vi "ListSharedResources.vi"(7 "exact name? (F: regex)":bool caption="exact", 8 "error in (no error)":errorcluster, 10 "Filter (regex|name)":string caption="Filter", 11 "SMO in":refnum<class "SMO.lvclass">) -> (0 "error out":errorcluster, 1 "resources found?":bool, 2 "Shared Resources":refnum<class "SMO.lvclass">[](array[class]), 3 "SMO out":refnum<class "SMO.lvclass">)   [LabVIEW 2021, in "smo.lvlib" / "SMO.lvclass"]
uses:
  SMO.lvclass
  SMO.lvclass/SMO.ctl
  Support/Attribute.Identity/Attribute.Identity.lvclass/Attribute.Identity.ctl
  Support/Attribute.Identity/Read GUID.vi
  Private/GetVariant(Attr).vi
  Support/Attribute.Identity/Read UniqueName.vi
  Private/ReftoDVR--SMO.vi
  Support/Attribute.Identity/Attribute.Identity.lvclass
  <vilib>/regexp/Match Regular Expression.xnode
  Registry/Registry-SMO.lvclass
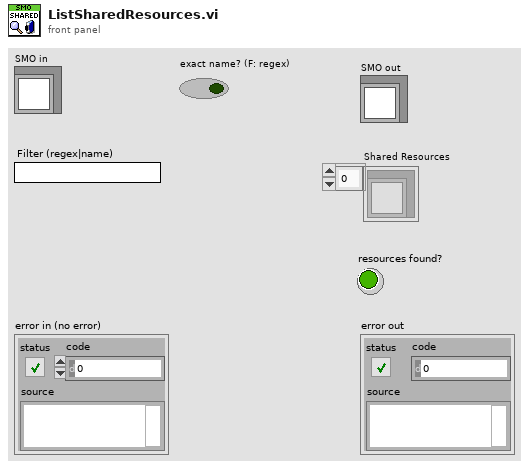
[diagram p1: front panel]
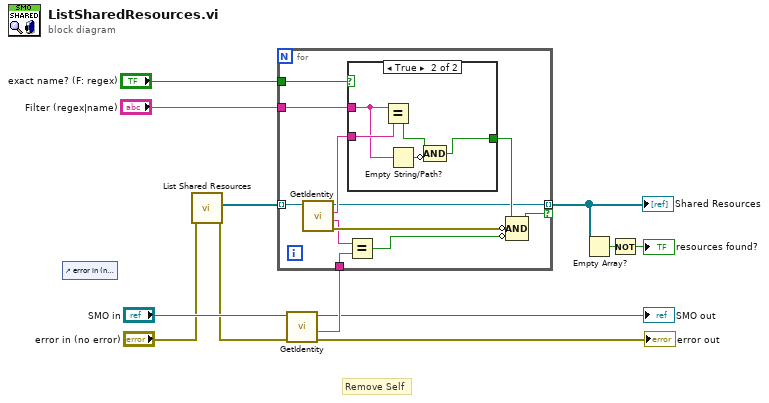
[diagram p0: block diagram]
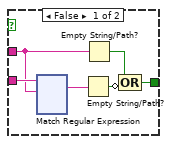
[diagram p2: hidden frame]
diagram:
  # "Remove Self"
  n1 = control-ref of="error in (no error)"() -> ()  [unwired: 1 out]
  n2 = call "List Shared Resources.vi"("error in (no error)"="error in (no error)") -> ("error out"=w1:errorcluster, "Shared Resources"=w3:refnum<class "SMO.lvclass">[])  [unwired: 9 in]
  n3 = call "GetIdentity.vi"("error in (no error)"=w1, "SMO in"="SMO in") -> ("error out"=→"error out":errorcluster, "GUID"=w7:string, "SMO out"=→"SMO out":refnum<class "SMO.lvclass">)  [unwired: 6 in, 1 out]
  n4 = for {
    tunnel: w3 -> [w23] mode=indexing
    tunnel: [w17] -> w11 mode=indexing if=w21
    tunnel: "Filter (regex|name)" -> [w18]
    tunnel: w7 -> [w14]
    tunnel: "exact name? (F: regex)" -> [w13]
    n5 = call "GetIdentity.vi"("SMO in"=w23) -> ("error out"=w20:errorcluster, "GUID"=w15:string, "Name"=w19:string, "SMO out"=w17:refnum<class "SMO.lvclass">)  [unwired: 7 in]
    n6 = Equal?(x=w15, y=w14) -> (x = y?=w16:bool)
    n7 = case shown="True" w13 {
      tunnel: [w29 w147] -> w22
      tunnel: w19 -> [w27 w151]
      tunnel: w18 -> [w24 w149]
      frame False {
        n8 = xnode "Match Regular Expression"("input string"=w27, "regular expression"=w24) -> ("whole match"=w26:string)  [unwired: 4 in, 4 out]
        n9 = Empty String/Path?(string/path=w26) -> (empty?=w25:bool)
        n10 = Empty String/Path?(string/path=w24) -> (empty?=w28:bool)
        n11 = Compound Arithmetic op=OR(w28, invert w25) -> (w29:bool)
      }
      frame True {
        n12 = Equal?(x=w149, y=w151) -> (x = y?=w148:bool)
        n13 = Empty String/Path?(string/path=w149) -> (empty?=w150:bool)
        n14 = Compound Arithmetic op=AND(w148, invert w150) -> (w147:bool)
      }
    }
    n15 = Compound Arithmetic op=AND(w22, invert w20, invert w16) -> (w21:bool)
  }
  "Shared Resources" <- w11
  n16 = Empty Array?(array=w11) -> (empty?=w10:bool)
  n17 = Not(x=w10) -> (.not. x?=→"resources found?":bool)
